vi "PI_WMS.vi"(8 "Pixels to reserve":i32, 9 "Axis":string, 10 "Position / Commandset":i32, 11 "Commandset in":string[](array[string])) -> (3 "Commandset out":string[](array[string]))   [LabVIEW 2009]
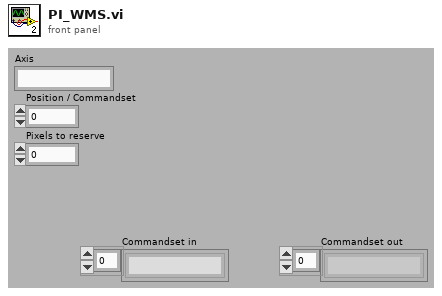
[diagram p1: front panel]
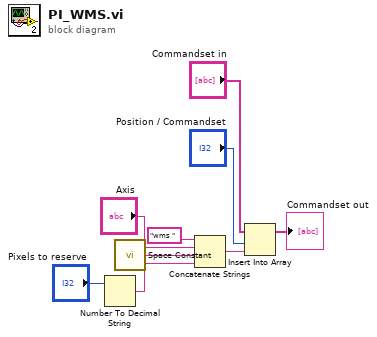
[diagram p0: block diagram]
diagram:
  n1 = Number To Decimal String(number="Pixels to reserve") -> (decimal integer string=w3:string)  [unwired: 1 out]
  n2 = call <vilib>:"Space Constant.vi"() -> ("String"=w4:string)
  n3 = Concatenate Strings("wms " ("string"), "Axis", w4, w3) -> (w7:string)
  n4 = Insert Into Array(array="Commandset in", index="Position / Commandset", new element=w7) -> (→"Commandset out":string[])
